vi "setRunToDocument.vi"(8 "error in (no error)":errorcluster, 11 "xwpfRun in":refnum<class "xwpfRun.lvclass">) -> (0 "error out":errorcluster, 3 "xwpfRun out":refnum<class "xwpfRun.lvclass">)   [LabVIEW 2017, in "Word_Specific.lvlib" / "xwpfRun.lvclass"]
uses:
  xwpfRun.lvclass
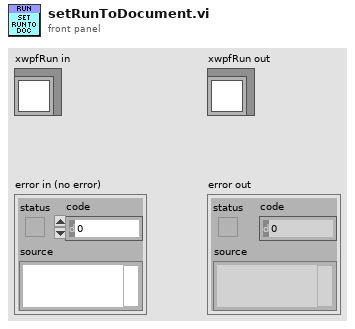
[diagram p1: front panel]
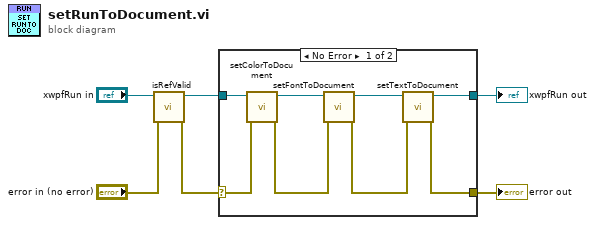
[diagram p0: block diagram]
diagram:
  n1 = call-dynamic "isRefValid.vi"("error in (no error)"="error in (no error)", "xwpfRun in"="xwpfRun in") -> ("error out"=w1:errorcluster, "xwpfRun out"=w3:refnum<class "xwpfRun.lvclass">)  [unwired: 8 in]
  n2 = case shown="No Error" w1 {
    selector: w1 -> [w10 w16]
    tunnel: [w7 w16] -> w6
    tunnel: [w11 w15] -> w4
    tunnel: w3 -> [w14 w15]
    frame No Error {
      n3 = call "setColorToDocument.vi"("error in (no error)"=w10, "xwpfRun in"=w14) -> ("error out"=w9:errorcluster, "xwpfRun out"=w13:refnum<class "xwpfRun.lvclass">)  [unwired: 8 in]
      n4 = call "setFontToDocument.vi"("error in (no error)"=w9, "xwpfRun in"=w13) -> ("error out"=w8:errorcluster, "xwpfRun out"=w12:refnum<class "xwpfRun.lvclass">)  [unwired: 8 in]
      n5 = call "setTextToDocument.vi"("error in (no error)"=w8, "xwpfRun in"=w12) -> ("error out"=w7:errorcluster, "xwpfRun out"=w11:refnum<class "xwpfRun.lvclass">)  [unwired: 8 in]
    }
    frame Error {
    }
  }
  "error out" <- w6
  "xwpfRun out" <- w4
